vi "Get State.vi"(8 "error in (no error)":errorcluster, 11 "NI-Scope Lock-in Driver in":refnum<class "NI-Scope Lock-in Driver.lvclass">) -> (0 "error out":errorcluster, 1 "Data ready":bool, 2 "Armed":bool, 3 "NI-Scope Lock-in Driver out":refnum<class "NI-Scope Lock-in Driver.lvclass">, 4 "Availiable Samples":u32, 5 "Finished":bool)   [LabVIEW 2016, in "NI-Scope Lock-in Driver.lvclass"]
uses:
  NI-Scope Lock-in Driver.lvclass
  NI-Scope Digitizer/Ni-Scope Digitizer.lvclass
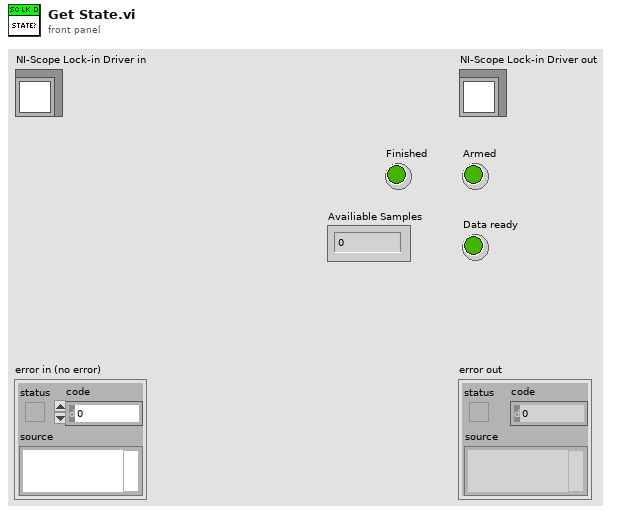
[diagram p1: front panel]
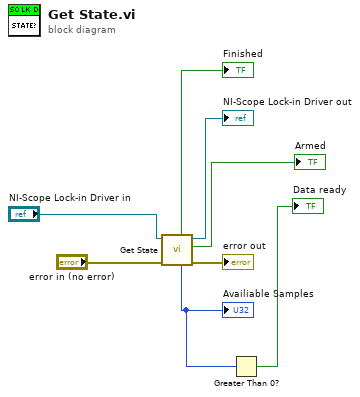
[diagram p0: block diagram]
diagram:
  n1 = call-parent "Get State.vi"("error in (no error)"="error in (no error)", "NI-Scope Digitizer in"="NI-Scope Lock-in Driver in") -> ("error out"=→"error out":errorcluster, "Armed"=→"Armed":bool, "NI-Scope Digitizer out"=→"NI-Scope Lock-in Driver out":refnum<class "NI-Scope Lock-in Driver.lvclass">, "Availiable Samples"=w2:u32, "Finished"=→"Finished":bool)  [unwired: 4 in, 1 out]
  "Availiable Samples" <- w2
  n2 = Greater Than 0?(x=w2) -> (x > 0?=→"Data ready":bool)
